vi "DASI_MS2000.vi"() -> (2 "error out":errorcluster)   [LabVIEW 2011]
panel:
  out "Value":string="12.3"
  out "command":string="stage.x.set"
  # "asi.port=com3\nas usual scale is meter!"
  # "noch nicht getestet\nnoch nicht stage.x.speed.set"
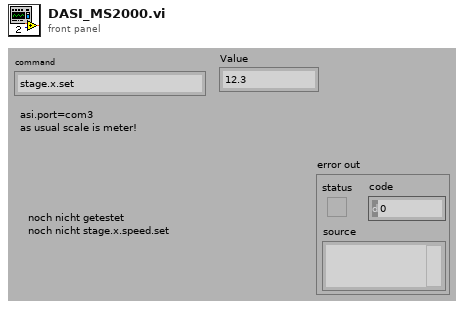
[diagram p1: front panel]
types:
  T1 = enum16{"None/#Datasets", "Clear", "TagValueOf#", "AddValues", "ReadValue", "ChangeValue", "Get all"}
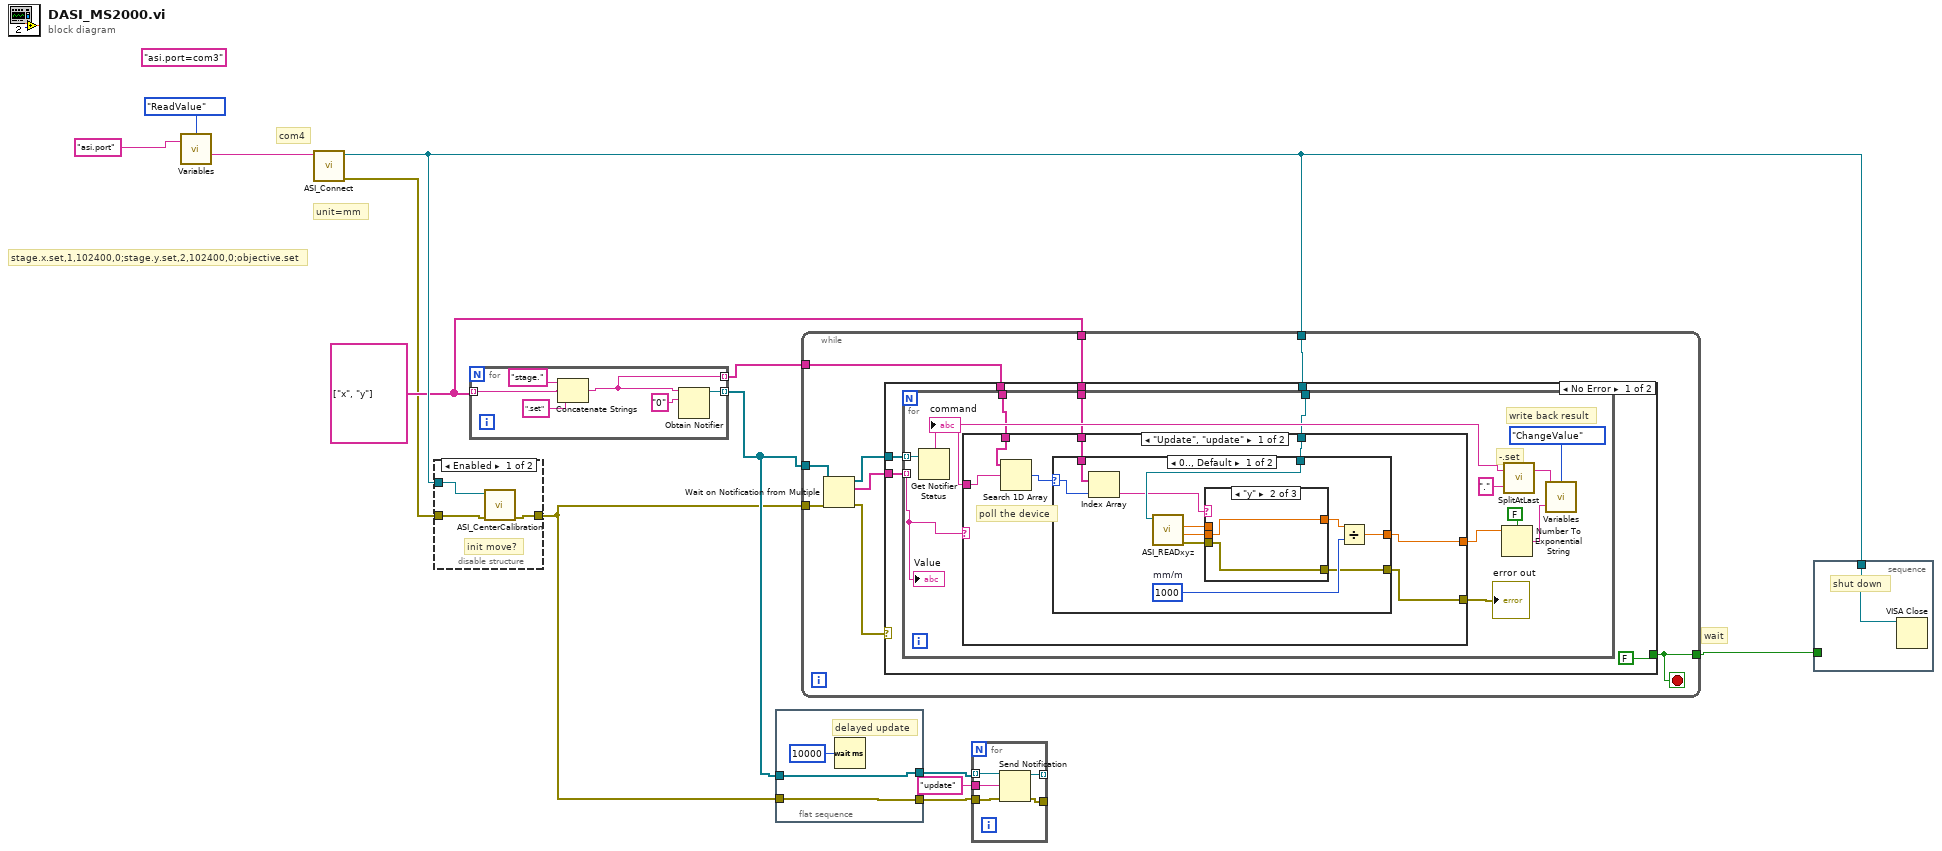
[diagram p0: block diagram]
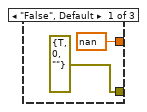
[diagram p3: hidden frame]
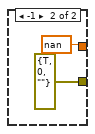
[diagram p5: hidden frame]
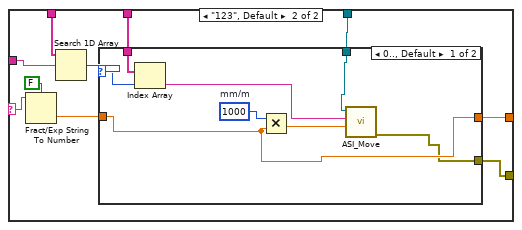
[diagram p6: hidden frame]
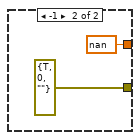
[diagram p7: hidden frame]
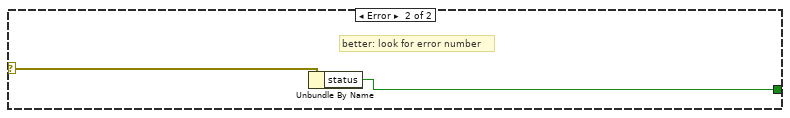
[diagram p8: hidden frame]
diagram:
  w2 = string[] ["x", "y"]
  (unwired) "asi.port=com3" ("Config-String")
  # "com4"
  # "stage.x.set,1,102400,0;stage.y.set,2,102400,0;objective.set"
  # "unit=mm"
  # "wait"
  n1 = call "Variables.vi"("Tag in"="asi.port", "Command"=T1."ReadValue") -> ("value out"=w5:string)  [unwired: 1 in, 2 out]
  n2 = call "ASI_Connect.vi"("VISA resource name"=w5) -> ("error out"=w1:errorcluster, "VISA resource name out"=w4:refnum<visa-resource-name>)  [unwired: 9 in]
  n3 = disable-structure shown="Enabled" {
    disable-tunnel: [w16 _] -> w6
    disable-tunnel: w4 -> [w15 _]
    disable-tunnel: w1 -> [w14 _]
    frame Enabled {
      # "init move?"
      n4 = call "ASI_CenterCalibration.vi"("error in (no error)"=w14, "VISA resource name"=w15) -> ("error out"=w16:errorcluster)  [unwired: 6 in, 3 out]
    }
    frame Disabled {
    }
  }
  n5 = for {
    tunnel: w2 -> [w18] mode=indexing
    tunnel: [w21] -> w9 mode=indexing
    tunnel: [w17] -> w3 mode=indexing
    n6 = Concatenate Strings("stage." ("string"), w18, ".set" ("string")) -> (w17:string)
    n7 = Obtain Notifier(name (unnamed)=w17, notification data type="0") -> (notifier out=w21:refnum<notifier>)  [unwired: 2 in, 2 out]
  }
  n8 = flat-sequence {
    tunnel: w9 -> [w24]
    tunnel: [w24] -> w8
    tunnel: w6 -> [w23]
    tunnel: [w23] -> w7
    frame #0 {
      # "delayed update"
      n9 = Wait (ms)(milliseconds to wait=u32 10000 ("Zu wartende ms")) -> ()  [unwired: 1 out]
    }
  }
  n10 = while {
    tunnel: w9 -> [w34]
    tunnel: w6 -> [w30]
    tunnel: [w29] -> w13
    tunnel: w4 -> [w28]
    tunnel: w3 -> [w27]
    tunnel: w2 -> [w26]
    stop <- w29 stop-if-true
    n11 = Wait on Notification from Multiple(0:w34, 3:w30) -> (8:w32:refnum<notifier>[], 9:w31:string[], 11:w33:errorcluster)  [unwired: 3 out]
    n12 = case shown="No Error" w33 {
      selector: w33 -> [_ w101]
      tunnel: w32 -> [w40 _]
      tunnel: w31 -> [w39 _]
      tunnel: [FALSE ("status") w100] -> w29
      tunnel: w28 -> [w37 _]
      tunnel: w27 -> [w36 _]
      tunnel: w26 -> [w35 _]
      frame No Error {
        n13 = for {
          tunnel: w40 -> [w51] mode=indexing
          tunnel: w39 -> [w46] mode=indexing
          tunnel: w37 -> [w43]
          tunnel: w36 -> [w42]
          tunnel: w35 -> [w41]
          # "write back result"
          # "-.set"
          n14 = Get Notifier Status(notifier=w51) -> (notifier name=w50:string)  [unwired: 1 in, 4 out]
          "command" <- w50
          n15 = case shown="\"Update\", \"update\"" w46 {
            selector: w46 -> [_ w88]
            tunnel: w50 -> [w59 w87]
            tunnel: [w56 w81] -> w48
            tunnel: [w55 w85] -> w47
            tunnel: w43 -> [w57 w82]
            tunnel: w42 -> [w60 w84]
            tunnel: w41 -> [w54 w80]
            frame "Update", "update" {
              # "poll the device"
              n16 = Search 1D Array(1D array=w60, element=w59) -> (index of element=w58:i32)  [unwired: 1 out]
              n17 = case shown="0.., Default" w58 {
                selector: w58 -> [w71 _]
                tunnel: [w61 errorcluster {"status"=TRUE, "code"=0, "source"=""} ("error in (no error)")] -> w55
                tunnel: w57 -> [w68 _]
                tunnel: [w70 nan] -> w56
                tunnel: w54 -> [w69 _]
                frame 0.., Default {
                  w67 = 1000  # mm/m
                  n18 = Index Array(array=w69, index=w71) -> (element=w66:string)
                  n19 = call "ASI_READxyz.vi"("VISA resource name"=w68) -> ("error out"=w62:errorcluster, "y [mm]"=w63:dbl, "x [mm]"=w65:dbl)  [unwired: 6 in, 2 out]
                  n20 = case shown="\"y\"" w66 {
                    tunnel: w65 -> [_ _ w77]
                    tunnel: [nan ("x [mm]") w75 w77] -> w64
                    tunnel: w63 -> [_ w75 _]
                    tunnel: w62 -> [_ w74 w76]
                    tunnel: [errorcluster {"status"=TRUE, "code"=0, "source"=""} ("error in (no error)") w74 w76] -> w61
                    frame "False", Default {
                    }
                    frame "y" {
                    }
                    frame "x" {
                    }
                  }
                  n21 = Divide(x=w64, y=w67) -> (x/y=w70:dbl)
                }
                frame -1 {
                }
              }
            }
            frame "123", Default {
              n22 = Fract/Exp String To Number(use system decimal point (T)=FALSE, string=w88) -> (number=w83:dbl)  [unwired: 3 out]
              n23 = Search 1D Array(1D array=w84, element=w87) -> (index of element=w86:i32)  [unwired: 1 out]
              n24 = case shown="0.., Default" w86 {
                selector: w86 -> [w97 _]
                tunnel: [w94 errorcluster {"status"=TRUE, "code"=0, "source"=""} ("error in (no error)")] -> w85
                tunnel: w83 -> [w96 _]
                tunnel: w82 -> [w95 _]
                tunnel: [w96 nan] -> w81
                tunnel: w80 -> [w91 _]
                frame 0.., Default {
                  w93 = 1000  # mm/m
                  n25 = Index Array(array=w91, index=w97) -> (element=w90:string)
                  n26 = Multiply(x=w93, y=w96) -> (x*y=w92:dbl)
                  n27 = call "ASI_Move.vi"("Position [mm]"=w92, "Axis"=w90, "VISA resource name"=w95) -> ("error out"=w94:errorcluster)  [unwired: 7 in, 1 out]
                }
                frame -1 {
                }
              }
            }
          }
          "error out" <- w47
          n28 = Number To Exponential String(number=w48, 1:FALSE ("use system decimal point (T)")) -> (E-format string=w53:string)  [unwired: 2 out]
          n29 = call "SplitAtLast.vi"("search char"=".", "In-String"=w50) -> ("Front (default)"=w45:string)  [unwired: 1 out]
          n30 = call "Variables.vi"("value"=w53, "Tag in"=w45, "Command"=T1."ChangeValue") -> ()  [unwired: 3 out]
          "Value" <- w46
        }
      }
      frame Error {
        # "better: look for error number"
        n31 = Unbundle By Name(w101) -> ("status"=w100:bool)
      }
    }
  }
  n32 = for {
    tunnel: w8 -> [w106] mode=indexing
    tunnel: w7 -> [w105]
    tunnel: [w104] -> _
    tunnel: [w103] -> _ mode=indexing
    tunnel: "update" -> [w102]
    n33 = Send Notification(notification=w102, notifier=w106, error in (no error)=w105) -> (notifier out=w103:refnum<notifier>, error out=w104:errorcluster)
  }
  n34 = stacked-sequence {
    tunnel: w13 -> [_]
    tunnel: w4 -> [w107]
    frame #0 {
      # "shut down"
      n35 = VISA Close(VISA resource name=w107) -> ()  [unwired: 1 in, 1 out]
    }
  }
